vi "Check TDMS File for Fragmentation.vi"() -> ()   [LabVIEW 2023]
doc: "This example demonstrates how to check data fragmentation in a .tdms file. By default, the file size of the .tdms file you want to check must be greater than 2MB. The <B>File Fragmented?</B> output returns TRUE if either of the following conditions occurs:\n* The ratio of the index file size to the .tdms file size is greater than 0.5.\n* The number of data segments in the .tdms file is greater than 100.\n\nRun this VI to check data fragmentation in your .tdms files. You can also modify the default input values of this VI. If the <B>File Fragmented?</B> returns TRUE, you can use the TDMS Defragment function to defragment the corresponding .tdms file."
panel:
  in  "Minimum Segment Count (100)":u64=100
  in  "Minimum Index to Main Ratio (0.5)":dbl=0.5 min=0.0 max=1.0 step=0.01
  in  "Minimum File Size (2MB)":u64=2
  out "File Fragmented?":bool
  # "Overview: Demonstrates how to check data fragmentation in a .tdms file.\nInstructions:\n1. Tune the three default input values to change your criteria for data fragmentation.\n2. Run this VI.\n3. Delete the .tdms file (located at [LabVIEW Data]\\Example Fragmented Data.tdms) when you are done."
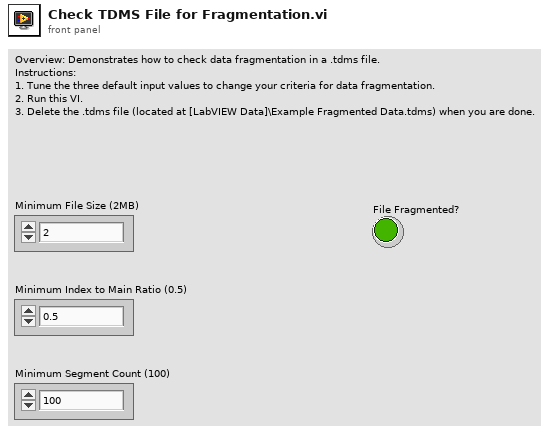
[diagram p1: front panel]
types:
  T1 = enum16{"open", "open or create", "create or replace", "create", "open (read-only)"}
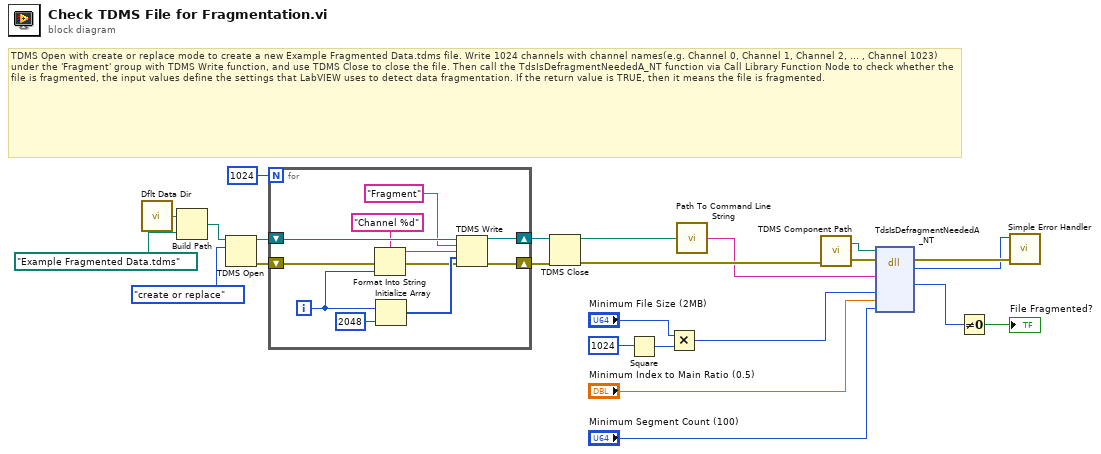
[diagram p0: block diagram]
diagram:
  # "TDMS Open with create or replace mode to create a new Example Fragmented Data.tdms file. Write 1024 channels with channel names(e.g. Channel 0, Channel 1, Channel 2, ... , Channel 1023) under the 'Fragment' group with TDMS Write function, and use TDMS Close to close the file. Then call the TdsIsDefragmentNeededA_NT function via Call Library Function Node to check whether the file is fragmented, the input values define the settings that LabVIEW uses to detect data fragmentation. If the return value is TRUE, then it means the file is fragmented."
  n1 = call <vilib>:"Dflt Data Dir.vi"() -> ("App:Default Data Directory"=w14:path)
  n2 = Build Path(base path=w14, name or relative path=path "Example Fragmented Data.tdms" ("file path")) -> (appended path=w11:path)
  n3 = TDMS Open(10:T1."create or replace" ("operation"), 11:w11) -> (0:w16:errorcluster, 3:w15:refnum<k34>)  [unwired: 5 in]
  n4 = for {
    N: 1024 -> [_]
    shift-right: [w34] -> w9
    shift-left: w15 -> [w35]
    shift-right: [w33] -> w10
    shift-left: w16 -> [w28]
    i -> [w31]
    n5 = Format Into String(format string="Channel %d", error in=w28, w31) -> (resulting string=w25:string, error out=w27:errorcluster)  [unwired: 1 in]
    n6 = Initialize Array(w31, 2048 ("dimension size")) -> (w30:i32[])
    n7 = TDMS Write(0:w35, 5:"Fragment" ("group name in (Untitled)"), 7:w25, 9:w30, 11:w27) -> (4:w34:refnum<k34>, 15:w33:errorcluster)  [unwired: 1 in, 2 out]
  }
  n8 = TDMS Close(8:w10, 11:w9) -> (0:w8:errorcluster, 3:w4:path)
  n9 = Square(x=u64 1024) -> (x^2=w22:u64)
  n10 = Multiply(x="Minimum File Size (2MB)", y=w22) -> (x*y=w5:u64)
  n11 = call <vilib>:"Path To Command Line String.vi"("path"=w4) -> ("string"=w3:string)
  n12 = call <vilib>:"TDMS Component Path.vi"("error in (no error)"=w8) -> ("error out"=w23:errorcluster, "appended path"=w24:path)  [unwired: 1 in]
  n13 = dll-call lib="?" fn="TdsIsDefragmentNeededA_NT" label="Is File Fragmented"(path in=w24, error in=w23, "filePath"=w3, "minMainFileSize"=w5, "minIndexToMainRatio"="Minimum Index to Main Ratio (0.5)", "minSegmentCount"="Minimum Segment Count (100)") -> (error out=w7:errorcluster, "return type"=w6:i32, "isFragmented"=w2:i32)  [unwired: 6 in, 1 out]
  n14 = Not Equal To 0?(x=w2) -> (x != 0?=→"File Fragmented?":bool)
  n15 = call <vilib>:"Simple Error Handler.vi"("error code (no error:0)"=w6, "error in (no error)"=w7) -> ()  [unwired: 1 in, 7 out]
